vi "DBL Multi-Array To Multi-Item Text.vi"(7 "Double Array":cluster{"Numeric Array":dbl[]}[](array[cluster])) -> (5 "Item Text":cluster{string[]}[](array[cluster]))   [LabVIEW 2019]
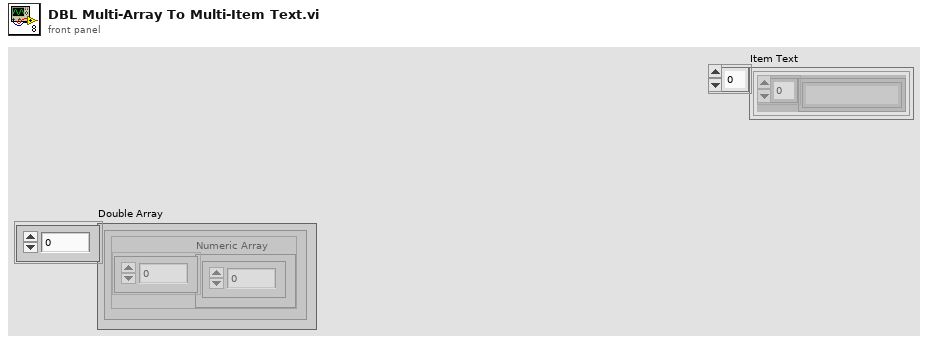
[diagram p1: front panel]
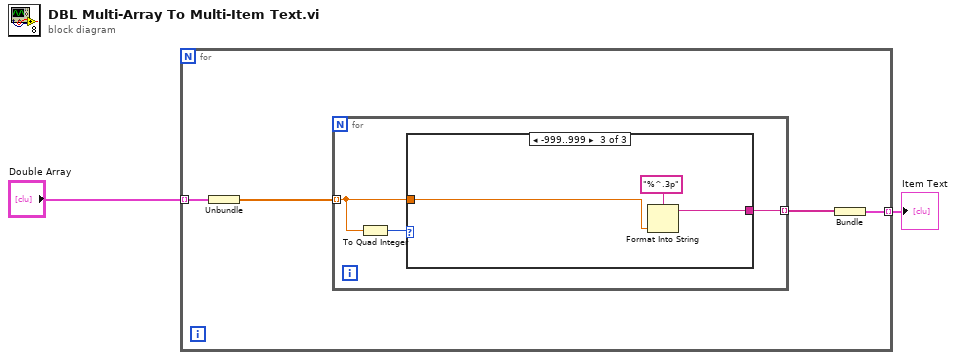
[diagram p0: block diagram]
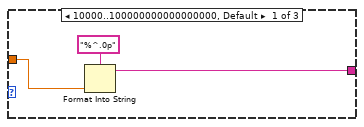
[diagram p2: hidden frame]
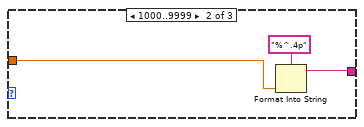
[diagram p3: hidden frame]
diagram:
  n1 = for {
    tunnel: "Double Array" -> [w5] mode=indexing
    tunnel: [w3] -> w1 mode=indexing
    n2 = Unbundle(w5) -> ("Numeric Array"=w6:dbl[])
    n3 = for {
      tunnel: w6 -> [w8] mode=indexing
      tunnel: [w9] -> w4 mode=indexing
      n4 = To Quad Integer(1:w8) -> (0:w7:i64)
      n5 = case shown="-999..999" w7 {
        tunnel: [w10 w14 w17] -> w9
        tunnel: w8 -> [w11 w13 w16]
        frame 10000..100000000000000000, Default {
          n6 = Format Into String(format string="%^.0p", w11) -> (resulting string=w10:string)  [unwired: 2 in, 1 out]
        }
        frame 1000..9999 {
          n7 = Format Into String(format string="%^.4p", w13) -> (resulting string=w14:string)  [unwired: 2 in, 1 out]
        }
        frame -999..999 {
          n8 = Format Into String(format string="%^.3p", w16) -> (resulting string=w17:string)  [unwired: 2 in, 1 out]
        }
      }
    }
    n9 = Bundle(w4) -> (w3:cluster{string[]})  [unwired: 1 in]
  }
  "Item Text" <- w1
